vi "Проект квадроКОПТЕР.vi"() -> ()   [LabVIEW 2013]
uses:
  <vilib>/Instr/_visa.llb/VISA Configure Serial Port (Instr).vi
  MadgwickOrientationFilter.lvlib
  <vilib>/picture/3D Picture Control/NI_3D Picture Control.lvlib
panel:
  out "Error 5":u8 caption="Error"
  in  "Tab Control":enum32{"3D", "Graphs", "U & I", "Out"}(tab)
  out "Scene Display":refnum<vi>(3d-picture)
  in  "x_y":dbl
  in  "z":dbl
  out "X":dbl
  out "Y":dbl
  out "Error":u8
  in  "VISA resource name":refnum<visa-resource-name>="COM5"
  out "Кватернион":T1(graph)
  out "высота":T1(graph)
  out "Q0":sgl
  out "Q1":sgl
  out "Q2":sgl
  out "Q3":sgl
  out "Boolean":bool
  out "Battery Voltage":dbl
  out "All Current":dbl
  out "Voltage":dbl(knob) scale=13.0..18.0
  out "Current":dbl(knob) scale=0.0..18.0
  out "Waveform Chart 3":T1(graph)
  in  "f_cut_diff_vel_xy":dbl
  in  "f_cut_diff_vel_xy b":bool
  in  "f_cut_err_vel_xy":dbl
  in  "f_cut_err_vel_xy b":bool
  in  "KP_Pos_xy b":bool
  in  "KP_Pos_xy":dbl
  in  "KP_Vel_xy b":bool
  in  "KP_Vel_xy":dbl
  in  "KD_Vel_xy":bool
  in  "KD_Vel_xy":dbl
  in  "KI_Acc_xy b":bool
  in  "KI_Vel_xy":dbl
  in  "f_cut_diff_vel_alt":dbl
  in  "f_cut_diff_vel_alt b":bool
  in  "f_cut_err_vel_alt":dbl
  in  "f_cut_diff_acc_alt b":bool
  in  "KI_ugol_z":dbl
  in  "KI_ugol_z_b":bool
  in  "KP_ugol_z":dbl
  in  "KP_ugol_z_b":bool
  in  "KI_rate_z":dbl
  in  "KI_vel_z_b":bool
  in  "KP_rate_z":dbl
  in  "KP_vel_z_b":bool
  in  "KD_rate_z":dbl
  in  "KD_vel_z_b":bool
  in  "KD_vel_xy_b":bool
  in  "KD_rate_xy":dbl
  in  "KI_vel_xy_b":bool
  in  "KP_vel_xy_b":bool
  in  "KI_rate_xy":dbl
  in  "KP_rate_xy":dbl
  in  "KI_ugla_xy_b":bool
  in  "KP_ugla_xy_b":bool
  in  "KI_ugla_xy":dbl
  in  "KP_ugla_xy":dbl
  in  "f_cut_diff":dbl
  in  "f_cut_diff_b":bool
  in  "KP_Pos_alt b":bool
  in  "KP_Pos_alt":dbl
  in  "KP_Vel_alt b":bool
  in  "KP_Vel_alt":dbl
  in  "KD_Vel_alt b":bool
  in  "KD_Vel_alt":dbl
  in  "KP_Acc_alt b":bool
  in  "KP_Acc_alt":dbl
  in  "KI_Acc_alt b":bool
  in  "KI_Vel_alt":dbl
  in  "KD_Acc_alt b":bool
  in  "KD_Acc_alt":dbl
  out "*(type *) &x 11":sgl
  out "*(type *) &x 10":sgl
  out "*(type *) &x 9":sgl
  out "*(type *) &x 8":sgl
  out "sqrt(x)":dbl
  out "unsigned byte array":u8[](array[numeric])
  out "String":string
  out "*(type *) &x 13":sgl
  out "*(type *) &x 12":sgl
  out "*(type *) &x 7":sgl
  out "*(type *) &x 6":sgl
  out "decimated array":u8[](array[numeric])
  out "*(type *) &x 5":sgl
  out "cluster":T1
  in  "stop":bool
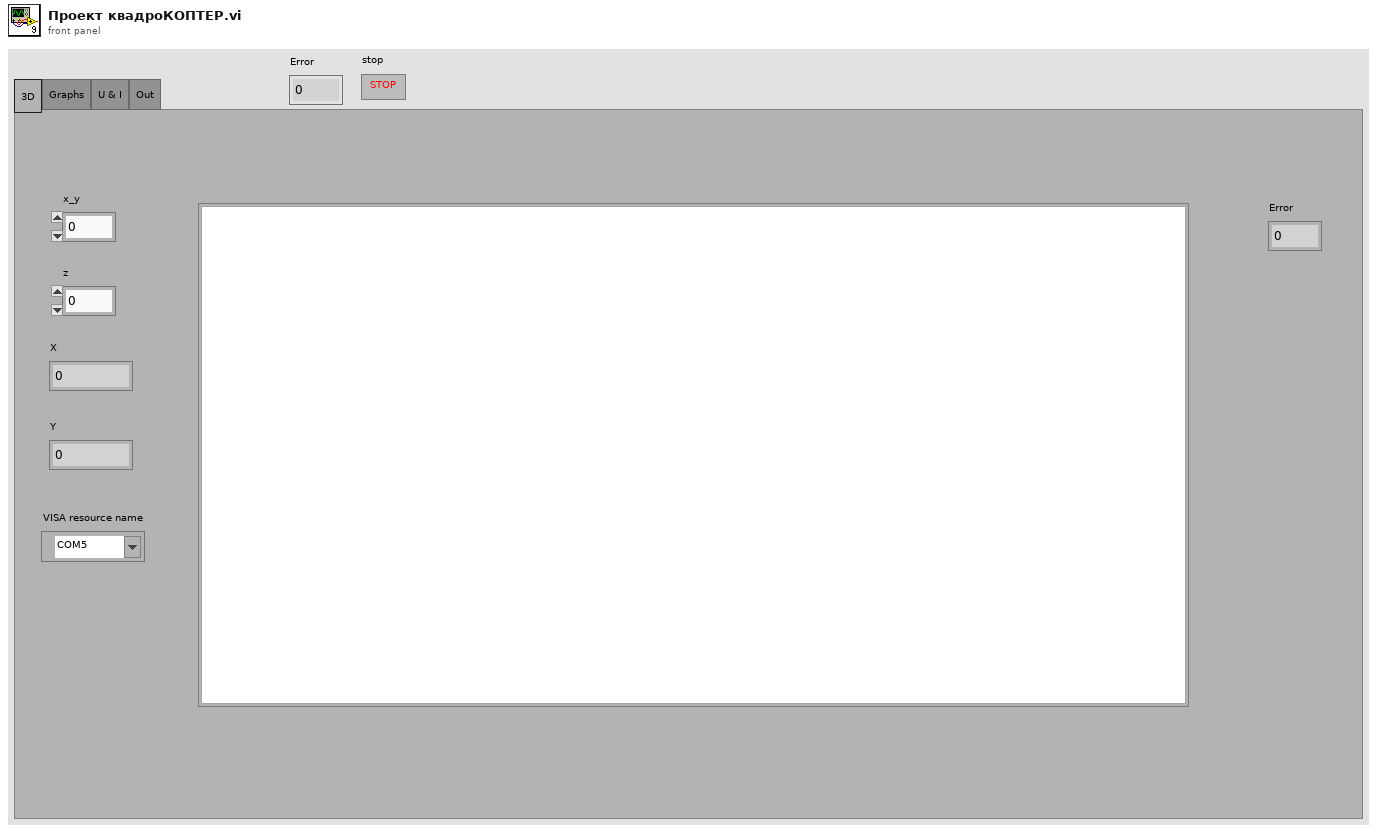
[diagram p1: front panel]
types:
  T1 = cluster{"[0]":dbl, "[1]":dbl, "[2]":dbl, "[3]":dbl, "[4]":dbl, "[5]":dbl, "[6]":dbl, "[7]":dbl, "[8]":dbl}
  T2 = enum16{"open", "replace", "create", "open or create", "replace or create", "replace or create with confirmation"}
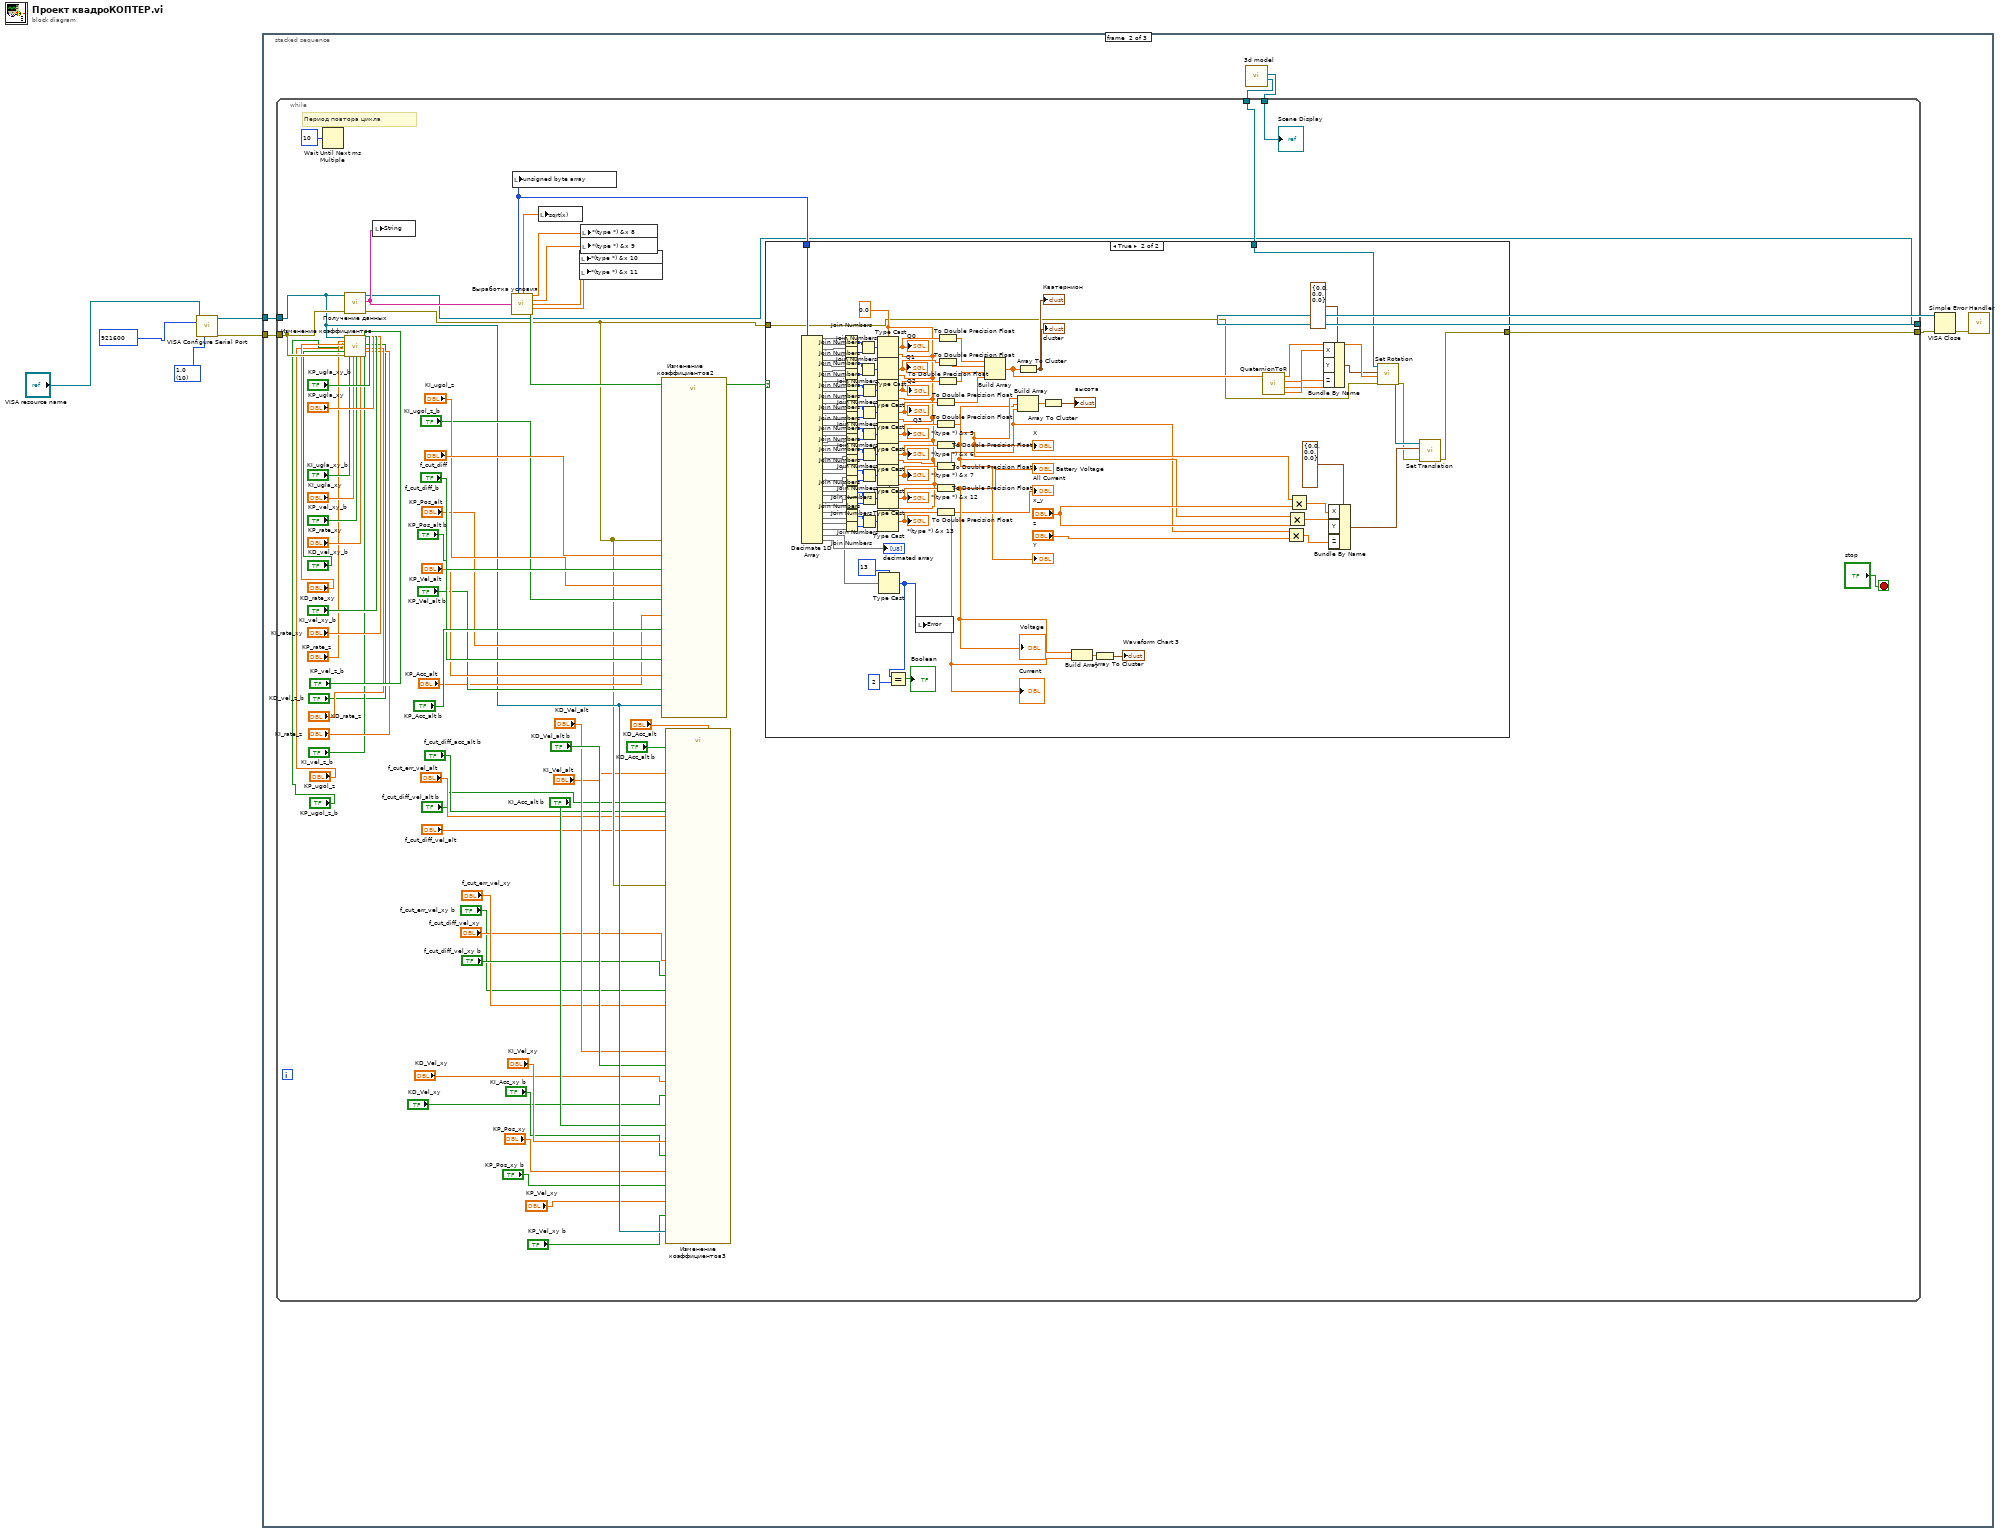
[diagram p0: block diagram]
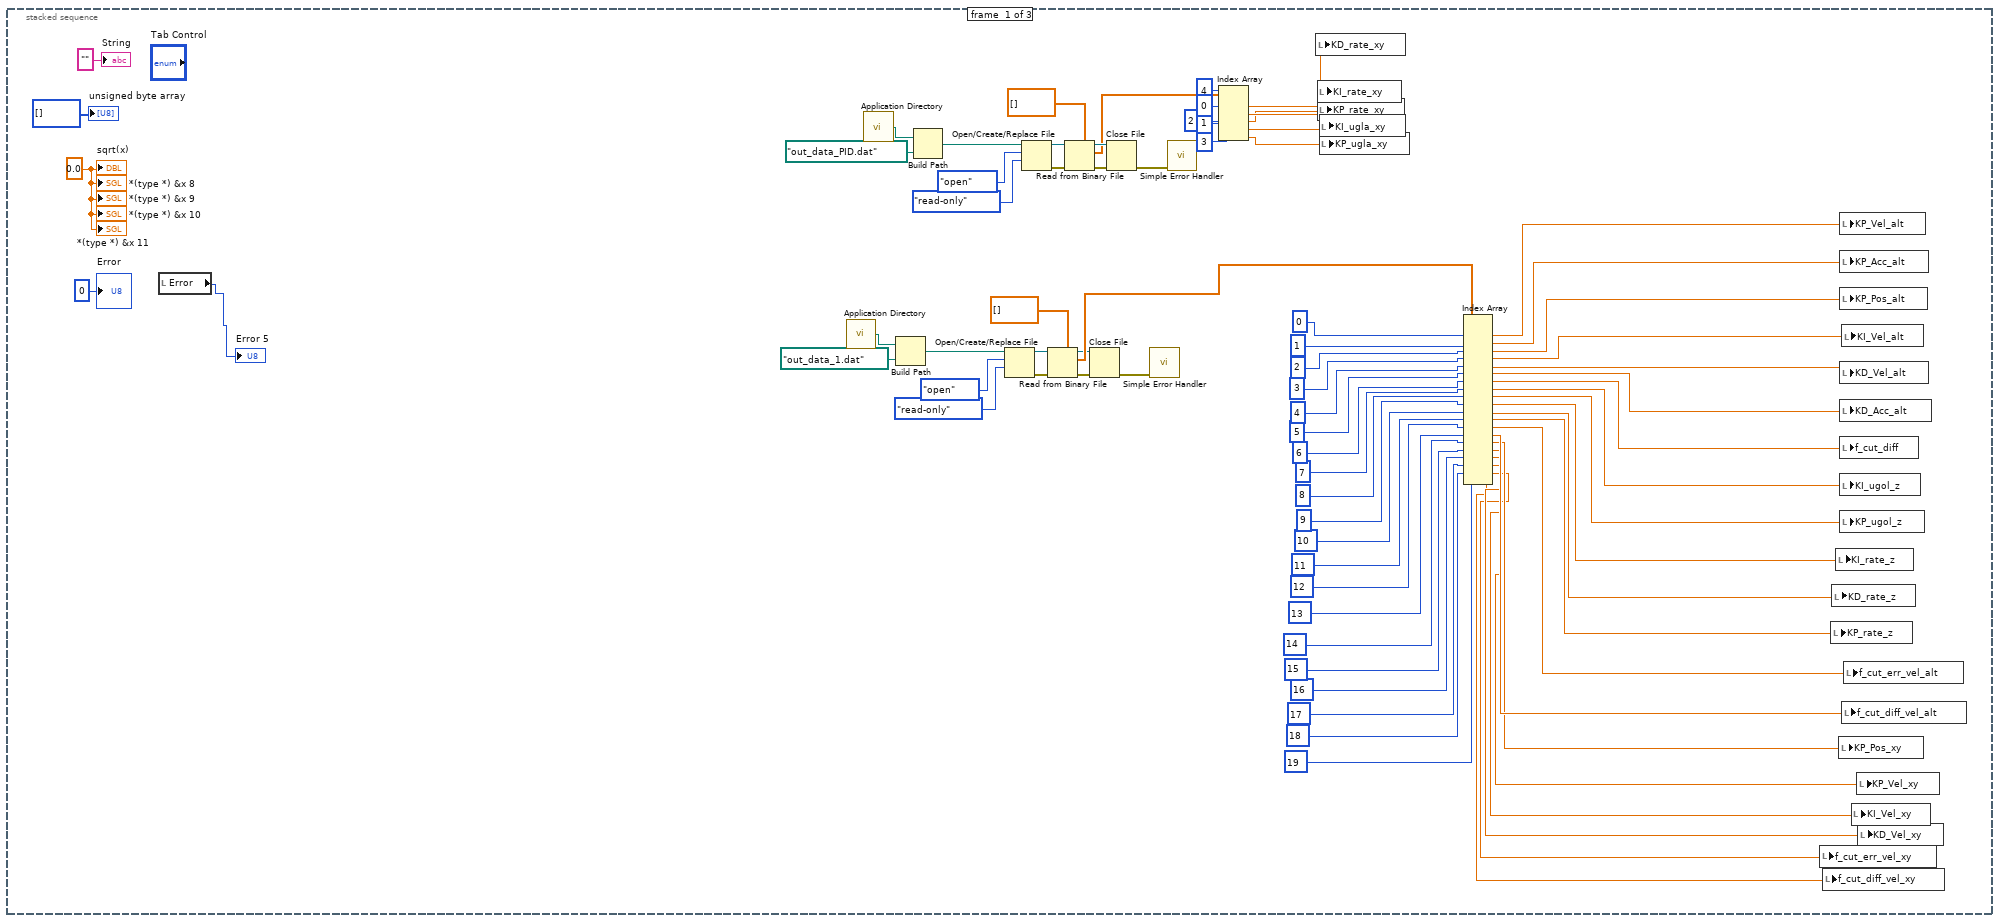
[diagram p2: hidden frame]
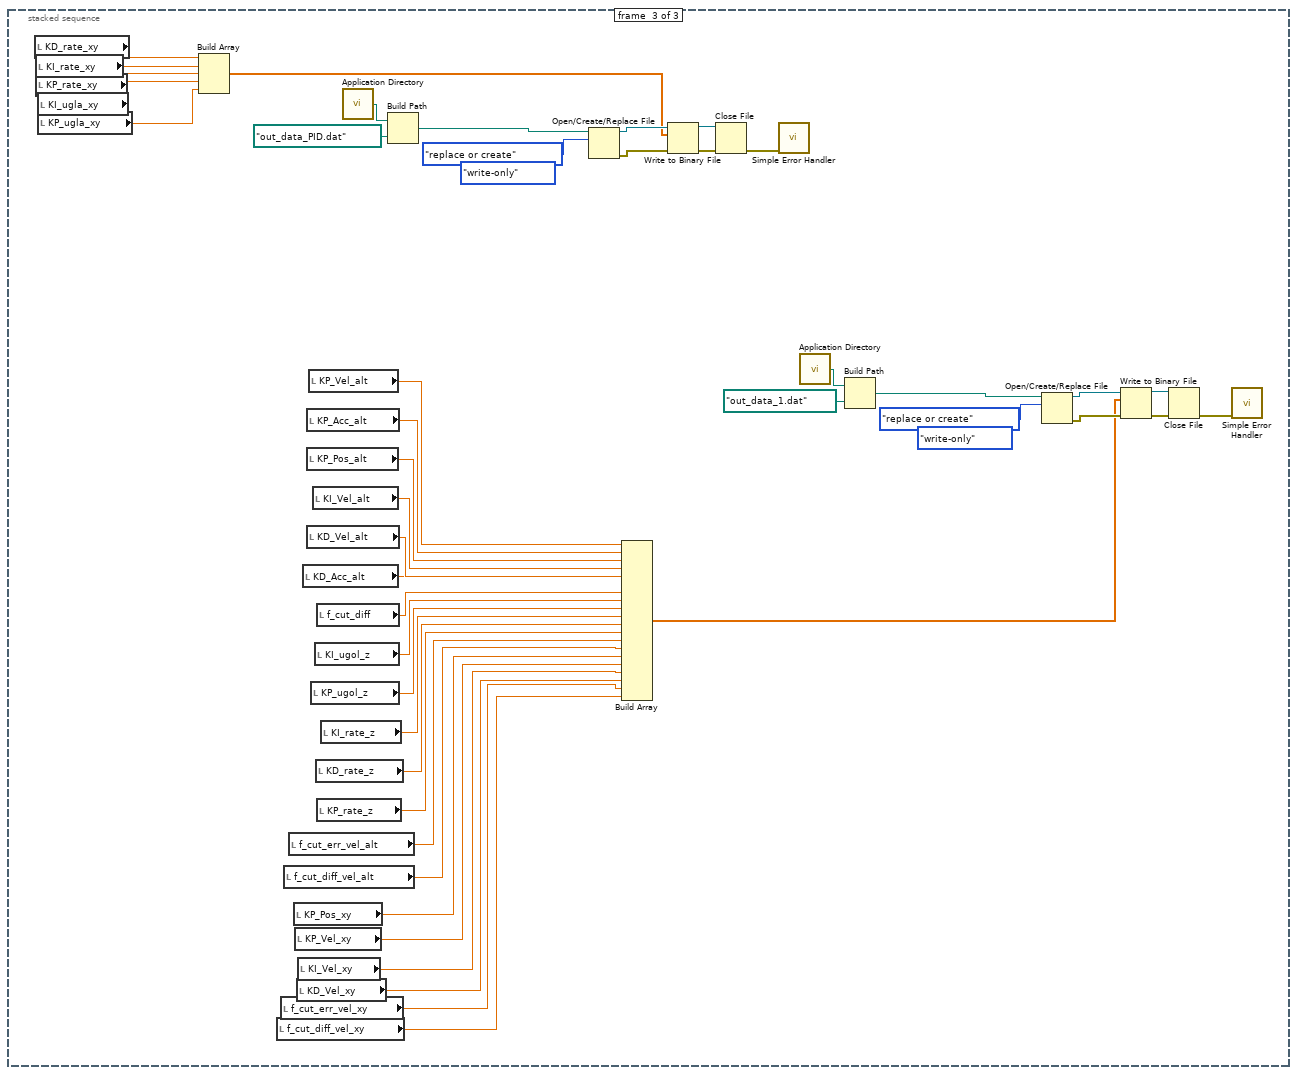
[diagram p4: hidden frame]
diagram:
  w3 = u16 10 items=["1.0"=10, "1.5"=15, "2.0"=20] ("stop bits (10: 1 bit)")
  n1 = call-poly "VISA Configure Serial Port"("VISA resource name"="VISA resource name", "baud rate (9600)"=u32 921600, "stop bits (10: 1 bit)"=w3) -> ("VISA resource name out"=w5:refnum<visa-resource-name>, "error out"=w4:errorcluster)  [unwired: 11 in]
  n2 = stacked-sequence {
    tunnel: w5 -> [_ w91 _]
    tunnel: w4 -> [_ w89 _]
    frame #0 {
      w82 = 0.0 ("sqrt(x)")
      n3 = local read "Error"() -> (→"Error 5":u8)
      n4 = call <vilib>:"Application Directory.vi"() -> ("Application Directory"=w56:path)
      n5 = call <vilib>:"Application Directory.vi"() -> ("Application Directory"=w74:path)
      n6 = Build Path(base path=w56, name or relative path=path "out_data_1.dat" ("default name")) -> (appended path=w52:path)
      n7 = Build Path(base path=w74, name or relative path=path "out_data_PID.dat" ("default name")) -> (appended path=w78:path)
      n8 = Open/Create/Replace File(file path (use dialog)=w52, operation (0:open)=T2."open", access (0:read/write)=enum16{"read/write", "read-only", "write-only"}."read-only") -> (refnum out=w57:refnum<file>, error out=w58:errorcluster)  [unwired: 3 in, 1 out]
      n9 = Open/Create/Replace File(file path (use dialog)=w78, operation (0:open)=T2."open", access (0:read/write)=enum16{"read/write", "read-only", "write-only"}."read-only") -> (refnum out=w73:refnum<file>, error out=w72:errorcluster)  [unwired: 3 in, 1 out]
      n10 = Read from Binary File(5:dbl[] [] ("appended array"), 8:w58, 11:w57) -> (0:w60:errorcluster, 2:w62:dbl[], 3:w59:refnum<file>)  [unwired: 3 in, 1 out]
      n11 = Read from Binary File(5:dbl[] [] ("appended array"), 8:w72, 11:w73) -> (0:w70:errorcluster, 2:w68:dbl[], 3:w71:refnum<file>)  [unwired: 3 in, 1 out]
      n12 = Close File(refnum=w59, error in=w60) -> (error out=w51:errorcluster)  [unwired: 1 out]
      n13 = Close File(refnum=w71, error in=w70) -> (error out=w79:errorcluster)  [unwired: 1 out]
      n14 = call <vilib>:"Simple Error Handler.vi"("error in (no error)"=w51) -> ()  [unwired: 4 in, 5 out]
      n15 = call <vilib>:"Simple Error Handler.vi"("error in (no error)"=w79) -> ()  [unwired: 4 in, 5 out]
      n16 = Index Array(array=w68, index #1=0 ("index"), index #2=1 ("index"), index #3=2 ("index"), index #4=3 ("index"), index #5=4 ("index")) -> (element #1=w50:dbl, element #2=w49:dbl, element #3=w48:dbl, element #4=w47:dbl, element #5=w46:dbl)
      n17 = local write "KD_rate_xy"(w50) -> ()
      n18 = local write "KI_rate_xy"(w49) -> ()
      n19 = local write "KP_rate_xy"(w48) -> ()
      n20 = local write "KI_ugla_xy"(w47) -> ()
      n21 = local write "KP_ugla_xy"(w46) -> ()
      n22 = Index Array(array=w62, index #1=0 ("index"), index #2=1 ("index"), index #3=2 ("index"), index #4=3 ("index"), index #5=4 ("index"), index #6=5 ("index"), index #7=6 ("index"), index #8=7 ("index"), index #9=8 ("index"), index #10=9 ("index"), index #11=10 ("index"), index #12=11 ("index"), index #13=12 ("index"), index #14=13 ("index"), index #15=14 ("index"), index #16=15 ("index"), index #17=16 ("index"), index #18=17 ("index"), index #19=18 ("index"), index #20=19 ("index")) -> (element #1=w45:dbl, element #2=w44:dbl, element #3=w43:dbl, element #4=w42:dbl, element #5=w41:dbl, element #6=w40:dbl, element #7=w39:dbl, element #8=w38:dbl, element #9=w37:dbl, element #10=w36:dbl, element #11=w35:dbl, element #12=w34:dbl, element #13=w19:dbl, element #14=w18:dbl, element #15=w11:dbl, element #16=w10:dbl, element #17=w9:dbl, element #18=w8:dbl, element #19=w7:dbl, element #20=w6:dbl)
      n23 = local write "f_cut_err_vel_xy"(w7) -> ()
      n24 = local write "f_cut_diff_vel_xy"(w6) -> ()
      n25 = local write "KP_rate_z"(w34) -> ()
      n26 = local write "KD_rate_z"(w35) -> ()
      n27 = local write "KI_rate_z"(w36) -> ()
      n28 = local write "KP_Pos_xy"(w11) -> ()
      n29 = local write "KP_Vel_alt"(w45) -> ()
      n30 = local write "KP_Acc_alt"(w44) -> ()
      n31 = local write "KP_Pos_alt"(w43) -> ()
      n32 = local write "KD_Vel_alt"(w41) -> ()
      n33 = local write "KD_Acc_alt"(w40) -> ()
      n34 = local write "f_cut_diff"(w39) -> ()
      n35 = local write "KI_ugol_z"(w38) -> ()
      n36 = local write "KP_ugol_z"(w37) -> ()
      n37 = local write "KI_Vel_alt"(w42) -> ()
      n38 = local write "f_cut_diff_vel_alt"(w18) -> ()
      n39 = local write "f_cut_err_vel_alt"(w19) -> ()
      n40 = local write "KI_Vel_xy"(w9) -> ()
      n41 = local write "KP_Vel_xy"(w10) -> ()
      n42 = local write "KD_Vel_xy"(w8) -> ()
      "String" <- "" ("String")
      "unsigned byte array" <- u8[] [] ("unsigned byte array")
      "sqrt(x)" <- w82
      "*(type *) &x 8" <- w82
      "*(type *) &x 9" <- w82
      "*(type *) &x 10" <- w82
      "*(type *) &x 11" <- w82
      "Error" <- u8 0 ("Error")
    }
    frame #1 {
      n43 = call "3d model.vi"() -> ("Коптер + оси"=w86:refnum<vi>, "Вся сцена"=w87:refnum<vi>)  [unwired: 9 in, 1 out]
      n44 = while {
        tunnel: w91 -> [w115]
        tunnel: [w126] -> w90
        tunnel: w89 -> [w155]
        tunnel: [w145] -> w88
        tunnel: w87 -> [w156]
        tunnel: w86 -> [w154]
        stop <- "stop" stop-if-true
        # "Период повтора цикла"
        n45 = Wait Until Next ms Multiple(millisecond multiple=u32 10) -> ()  [unwired: 1 out]
        n46 = call "Получение данных.vi"("error in (no error)"=w155, "VISA Refnum in"=w115) -> ("error out"=w114:errorcluster, "String"=w152:string, "VISA Refnum out"=w126:refnum<visa-resource-name>)  [unwired: 7 in]
        n47 = call "Изменение коэффициентов.vi"("VISA Refnum in"=w115, "KP_ugol_z"="KP_ugol_z", "KD_vel"="KD_rate_xy", "KP_ugol_z_b"="KP_ugol_z_b", "KD_vel 2"="KD_vel_xy_b", "error in (no error)"=w155, "KI_vel 2"="KI_vel_xy_b", "KI_ugla 2"="KI_ugla_xy_b", "KP_ugla"="KP_ugla_xy", "KI_ugla"="KI_ugla_xy", "KP_ugla 2"="KP_ugla_xy_b", "KP_vel 2"="KP_vel_xy_b", "KI_vel"="KI_rate_xy", "KP_vel"="KP_rate_xy", "KP_vel_z_b"="KP_vel_z_b", "KP_vel_z"="KP_rate_z", "KD_vel_z_b"="KD_vel_z_b", "KD_vel_z"="KD_rate_z", "KI_vel_z"="KI_rate_z", "KI_vel_z_b"="KI_vel_z_b") -> ()
        n48 = local write "String"(w152) -> ()
        n49 = call "Выработка условия.vi"("String"=w152) -> ("unsigned byte array"=w151:u8[], "sqrt(x)"=w150:dbl, "*(type *) &x 8"=w149:sgl, "*(type *) &x 9"=w148:sgl, "*(type *) &x 10"=w147:sgl, "*(type *) &x 11"=w146:sgl, "Boolean"=w153:bool)  [unwired: 8 in]
        n50 = local write "unsigned byte array"(w151) -> ()
        n51 = local write "sqrt(x)"(w150) -> ()
        n52 = local write "*(type *) &x 10"(w147) -> ()
        n53 = local write "*(type *) &x 11"(w146) -> ()
        n54 = local write "*(type *) &x 8"(w149) -> ()
        n55 = local write "*(type *) &x 9"(w148) -> ()
        n56 = call "Изменение коэффициентов2.vi"("KI_ugol_z_b"="KI_ugol_z_b", "KI_ugol_z"="KI_ugol_z", "f_cut_diff_b"="f_cut_diff_b", "f_cut_diff"="f_cut_diff", "KP_Pos_alt b"="KP_Pos_alt b", "KP_Pos_alt"="KP_Pos_alt", "KP_Vel_alt b"="KP_Vel_alt b", "KP_Vel_alt"="KP_Vel_alt", "VISA Refnum in"=w115, "error in (no error)"=w114, "KP_Acc_alt b"="KP_Acc_alt b", "KP_Acc_alt"="KP_Acc_alt") -> ()  [unwired: 16 in]
        n57 = call "Изменение коэффициентов3.vi"("VISA Refnum in"=w115, "error in (no error)"=w114, "f_cut_diff_vel_xy b"="f_cut_diff_vel_xy b", "KP_Pos_xy b"="KP_Pos_xy b", "KD_Vel_alt b"="KD_Vel_alt b", "KD_Vel_alt"="KD_Vel_alt", "f_cut_err_vel_xy"="f_cut_err_vel_xy", "KI_Acc_alt b"="KI_Acc_alt b", 8:"KD_Vel_xy"="KD_Vel_xy", "KP_Pos_xy"="KP_Pos_xy", "f_cut_err_vel_xy b"="f_cut_err_vel_xy b", "f_cut_diff_vel_xy"="f_cut_diff_vel_xy", 12:"KD_Vel_xy"="KD_Vel_xy", "KP_Vel_xy b"="KP_Vel_xy b", "KI_Vel_xy"="KI_Vel_xy", "f_cut_diff_vel_alt"="f_cut_diff_vel_alt", "KI_Vel_xy b"="KI_Acc_xy b", "f_cut_diff_vel_alt b"="f_cut_diff_vel_alt b", "KI_Acc_alt"="KI_Vel_alt", "KD_Acc_alt b"="KD_Acc_alt b", "KP_Vel_xy"="KP_Vel_xy", "KD_Acc_alt"="KD_Acc_alt", "f_cut_diff_acc_alt b"="f_cut_diff_acc_alt b", "f_cut_diff_acc_alt"="f_cut_err_vel_alt") -> ()  [unwired: 4 in]
        n58 = case shown="True" w153 {
          tunnel: w151 -> [_ w223]
          tunnel: w154 -> [_ w167]
          tunnel: w114 -> [w159 w166]
          tunnel: [w159 w164] -> w145
          frame False {
          }
          frame True {
            w176 = sgl 0.0
            n59 = Decimate 1D Array(w223) -> (w231:u8[], w232:u8[], w233:u8[], w234:u8[], w239:u8[], w240:u8[], w241:u8[], w242:u8[], w247:u8[], w248:u8[], w249:u8[], w250:u8[], w251:u8[], w252:u8[], w253:u8[], w254:u8[], w266:u8[], w267:u8[], w268:u8[], w269:u8[], w214:u8[], w213:u8[], w212:u8[], w211:u8[], w210:u8[], w209:u8[], w208:u8[], w207:u8[], w189:u8[], w188:u8[], w187:u8[], w186:u8[], w180:u8[], w179:u8[], w178:u8[], w177:u8[], w175:u8[], →"decimated array":u8[])
            n60 = Join Numbers(hi=w231, lo=w232) -> ((hi.lo)=w235:u16[])
            n61 = Join Numbers(hi=w233, lo=w234) -> ((hi.lo)=w236:u16[])
            n62 = Join Numbers(hi=w239, lo=w240) -> ((hi.lo)=w237:u16[])
            n63 = Join Numbers(hi=w241, lo=w242) -> ((hi.lo)=w238:u16[])
            n64 = Join Numbers(hi=w247, lo=w248) -> ((hi.lo)=w243:u16[])
            n65 = Join Numbers(hi=w249, lo=w250) -> ((hi.lo)=w244:u16[])
            n66 = Join Numbers(hi=w251, lo=w252) -> ((hi.lo)=w245:u16[])
            n67 = Join Numbers(hi=w253, lo=w254) -> ((hi.lo)=w246:u16[])
            n68 = Join Numbers(hi=w266, lo=w267) -> ((hi.lo)=w263:u16[])
            n69 = Join Numbers(hi=w268, lo=w269) -> ((hi.lo)=w264:u16[])
            n70 = Join Numbers(hi=w214, lo=w213) -> ((hi.lo)=w219:u16[])
            n71 = Join Numbers(hi=w212, lo=w211) -> ((hi.lo)=w220:u16[])
            n72 = Join Numbers(hi=w210, lo=w209) -> ((hi.lo)=w215:u16[])
            n73 = Join Numbers(hi=w208, lo=w207) -> ((hi.lo)=w216:u16[])
            n74 = Join Numbers(hi=w189, lo=w188) -> ((hi.lo)=w190:u16[])
            n75 = Join Numbers(hi=w187, lo=w186) -> ((hi.lo)=w191:u16[])
            n76 = Join Numbers(hi=w180, lo=w179) -> ((hi.lo)=w181:u16[])
            n77 = Join Numbers(hi=w178, lo=w177) -> ((hi.lo)=w182:u16[])
            n78 = Join Numbers(hi=w235, lo=w236) -> ((hi.lo)=w255:u32[])
            n79 = Join Numbers(hi=w237, lo=w238) -> ((hi.lo)=w202:u32[])
            n80 = Join Numbers(hi=w243, lo=w244) -> ((hi.lo)=w257:u32[])
            n81 = Join Numbers(hi=w245, lo=w246) -> ((hi.lo)=w258:u32[])
            n82 = Join Numbers(hi=w263, lo=w264) -> ((hi.lo)=w265:u32[])
            n83 = Join Numbers(hi=w219, lo=w220) -> ((hi.lo)=w221:u32[])
            n84 = Join Numbers(hi=w215, lo=w216) -> ((hi.lo)=w217:u32[])
            n85 = Join Numbers(hi=w190, lo=w191) -> ((hi.lo)=w192:u32[])
            n86 = Join Numbers(hi=w181, lo=w182) -> ((hi.lo)=w183:u32[])
            n87 = Type Cast(type=w176, x=w255) -> (*(type *) &x=w198:sgl)
            "Q0" <- w198
            n88 = Type Cast(type=w176, x=w202) -> (*(type *) &x=w199:sgl)
            "Q1" <- w199
            n89 = Type Cast(type=w176, x=w257) -> (*(type *) &x=w200:sgl)
            "Q2" <- w200
            n90 = Type Cast(type=w176, x=w258) -> (*(type *) &x=w201:sgl)
            "Q3" <- w201
            n91 = Type Cast(type=w176, x=w265) -> (*(type *) &x=w272:sgl)
            "*(type *) &x 5" <- w272
            n92 = Type Cast(type=w176, x=w221) -> (*(type *) &x=w222:sgl)
            "*(type *) &x 6" <- w222
            n93 = Type Cast(type=w176, x=w217) -> (*(type *) &x=w218:sgl)
            "*(type *) &x 7" <- w218
            n94 = Type Cast(type=w176, x=w192) -> (*(type *) &x=w185:sgl)
            "*(type *) &x 12" <- w185
            n95 = Type Cast(type=w176, x=w183) -> (*(type *) &x=w184:sgl)
            "*(type *) &x 13" <- w184
            n96 = Type Cast(type=u8 13 ("y"), x=w175) -> (*(type *) &x=w163:u8)
            n97 = Equal?(x=w163, y=u8 2) -> (x = y?=→"Boolean":bool)
            n98 = local write "Error"(w163) -> ()
            n99 = To Double Precision Float(number=w201) -> (double precision float=w261:dbl)
            n100 = To Double Precision Float(number=w272) -> (double precision float=w162:dbl)
            "X" <- w162
            n101 = To Double Precision Float(number=w222) -> (double precision float=w161:dbl)
            "Y" <- w161
            n102 = To Double Precision Float(number=w218) -> (double precision float=w160:dbl)
            n103 = To Double Precision Float(number=w185) -> (double precision float=w169:dbl)
            "Battery Voltage" <- w169
            "Voltage" <- w169
            n104 = To Double Precision Float(number=w184) -> (double precision float=w168:dbl)
            "All Current" <- w168
            "Current" <- w168
            n105 = To Double Precision Float(number=w198) -> (double precision float=w256:dbl)
            n106 = To Double Precision Float(number=w199) -> (double precision float=w259:dbl)
            n107 = To Double Precision Float(number=w200) -> (double precision float=w260:dbl)
            n108 = Build Array(w256, w259, w260, w261) -> (w262:dbl[])
            n109 = Build Array(w162, w161, w160) -> (w206:dbl[])
            n110 = Array To Cluster(array=w262) -> (cluster=→"Кватернион" →"cluster":T1)
            n111 = Array To Cluster(array=w206) -> (cluster=→"высота":T1)
            n112 = Build Array(w169, w168) -> (w171:dbl[])
            n113 = Array To Cluster(array=w171) -> (cluster=→"Waveform Chart 3":T1)
            n114 = call "QuaternionToR.vi"("Quaternion"=w262) -> ("Rz"=w227:dbl, "Ry"=w226:dbl, "Rx"=w225:dbl, "Theta"=w230:dbl)  [unwired: 7 in]
            n115 = Multiply(x=w160, y="z") -> (x*y=w195:dbl)
            n116 = Multiply(x=w161, y="x_y") -> (x*y=w196:dbl)
            n117 = Multiply(x=w162, y="x_y") -> (x*y=w194:dbl)
            n118 = Bundle By Name(cluster=cluster{"X":sgl, "Y":sgl, "Z":sgl} {"X"=0.0, "Y"=0.0, "Z"=0.0} ("Axis"), "X"=w225, "Y"=w226, "Z"=w227) -> (w228:cluster{"X":sgl, "Y":sgl, "Z":sgl})
            n119 = Bundle By Name(cluster=cluster{"X":sgl, "Y":sgl, "Z":sgl} {"X"=0.0, "Y"=0.0, "Z"=0.0} ("Axis"), "X"=w194, "Y"=w196, "Z"=w195) -> (w270:cluster{"X":sgl, "Y":sgl, "Z":sgl})
            n120 = call <vilib>:"Set Rotation.vi"("error in (no error)"=w166, "Angle"=w230, "Axis"=w228, "Scene Object"=w167) -> ("error out"=w165:errorcluster, "Rotated Scene Object"=w197:refnum<vi>)  [unwired: 6 in]
            n121 = call <vilib>:"Set Translation.vi"("error in (no error)"=w165, "Translation"=w270, "Scene Object"=w197) -> ("error out"=w164:errorcluster)  [unwired: 7 in, 1 out]
          }
        }
        "Scene Display" <- w156
      }
      n122 = VISA Close(VISA resource name=w90, error in (no error)=w88) -> (error out=w85:errorcluster)
      n123 = call <vilib>:"Simple Error Handler.vi"("error in (no error)"=w85) -> ()  [unwired: 4 in, 5 out]
    }
    frame #2 {
      (unwired) enum16{"read/write", "read-only", "write-only"}."write-only" ("access (0:read/write)")
      (unwired) enum16{"read/write", "read-only", "write-only"}."write-only" ("access (0:read/write)")
      n124 = local read "KD_rate_xy"() -> (w317:dbl)
      n125 = local read "KI_rate_xy"() -> (w316:dbl)
      n126 = local read "KP_rate_xy"() -> (w315:dbl)
      n127 = local read "KI_ugla_xy"() -> (w314:dbl)
      n128 = local read "KP_ugla_xy"() -> (w313:dbl)
      n129 = Build Array(w317, w316, w315, w314, w313) -> (w303:dbl[])
      n130 = local read "f_cut_diff_vel_xy"() -> (w273:dbl)
      n131 = local read "f_cut_err_vel_xy"() -> (w274:dbl)
      n132 = local read "f_cut_diff_vel_alt"() -> (w279:dbl)
      n133 = local read "f_cut_err_vel_alt"() -> (w280:dbl)
      n134 = local read "KP_Pos_xy"() -> (w278:dbl)
      n135 = local read "KP_Vel_xy"() -> (w277:dbl)
      n136 = local read "KD_Vel_xy"() -> (w275:dbl)
      n137 = local read "KI_Vel_xy"() -> (w276:dbl)
      n138 = local read "KD_Acc_alt"() -> (w288:dbl)
      n139 = local read "KP_Acc_alt"() -> (w292:dbl)
      n140 = local read "KP_Pos_alt"() -> (w291:dbl)
      n141 = local read "KD_Vel_alt"() -> (w289:dbl)
      n142 = local read "KP_Vel_alt"() -> (w293:dbl)
      n143 = local read "KP_ugol_z"() -> (w285:dbl)
      n144 = local read "KI_Vel_alt"() -> (w290:dbl)
      n145 = local read "KI_ugol_z"() -> (w286:dbl)
      n146 = local read "KD_rate_z"() -> (w283:dbl)
      n147 = local read "f_cut_diff"() -> (w287:dbl)
      n148 = local read "KP_rate_z"() -> (w282:dbl)
      n149 = local read "KI_rate_z"() -> (w284:dbl)
      n150 = call <vilib>:"Application Directory.vi"() -> ("Application Directory"=w310:path)
      n151 = Build Path(base path=w310, name or relative path=path "out_data_PID.dat" ("default name")) -> (appended path=w312:path)
      n152 = Open/Create/Replace File(file path (use dialog)=w312, operation (0:open)=T2."replace or create") -> (refnum out=w305:refnum<file>, error out=w304:errorcluster)  [unwired: 4 in, 1 out]
      n153 = Build Array(w293, w292, w291, w290, w289, w288, w287, w286, w285, w284, w283, w282, w280, w279, w278, w277, w276, w275, w274, w273) -> (w281:dbl[])
      n154 = Write to Binary File(file (use dialog)=w305, data=w303, error in=w304) -> (refnum out=w306:refnum<file>, error out=w307:errorcluster)  [unwired: 3 in, 1 out]
      n155 = Close File(refnum=w306, error in=w307) -> (error out=w308:errorcluster)  [unwired: 1 out]
      n156 = call <vilib>:"Simple Error Handler.vi"("error in (no error)"=w308) -> ()  [unwired: 4 in, 5 out]
      n157 = call <vilib>:"Application Directory.vi"() -> ("Application Directory"=w296:path)
      n158 = Build Path(base path=w296, name or relative path=path "out_data_1.dat" ("default name")) -> (appended path=w294:path)
      n159 = Open/Create/Replace File(file path (use dialog)=w294, operation (0:open)=T2."replace or create") -> (refnum out=w301:refnum<file>, error out=w302:errorcluster)  [unwired: 4 in, 1 out]
      n160 = Write to Binary File(file (use dialog)=w301, data=w281, error in=w302) -> (refnum out=w300:refnum<file>, error out=w299:errorcluster)  [unwired: 3 in, 1 out]
      n161 = Close File(refnum=w300, error in=w299) -> (error out=w298:errorcluster)  [unwired: 1 out]
      n162 = call <vilib>:"Simple Error Handler.vi"("error in (no error)"=w298) -> ()  [unwired: 4 in, 5 out]
    }
  }
